vi "Init.vi"(0 "Experiment2D in":refnum<class "Experiment2D.lvclass">, 5 "Path":path=path "C:/Users/Sergei/Documents", 7 "Measurement2D.lvclass":refnum<class "Measurement2D.lvclass">, 9 "Data2D.lvclass":refnum<class "Data2D.lvclass">, 11 "error in (no error)":errorcluster) -> (4 "Experiment2D out":refnum<class "Experiment2D.lvclass">, 15 "error out":errorcluster)   [LabVIEW 2014, in "Experiment2D.lvclass"]
uses:
  Experiment2D.lvclass
  Measurement/Measurement2D/Measurement2D.lvclass
  Instrument/Instrument/Instrument.lvclass
  Data/Data2D/Data2D.lvclass
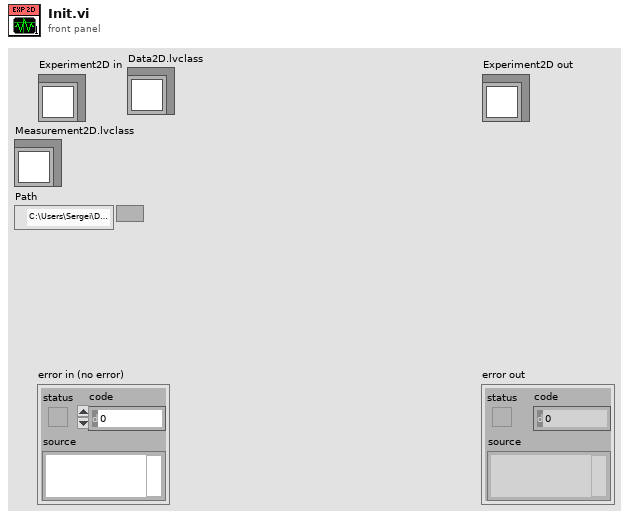
[diagram p1: front panel]
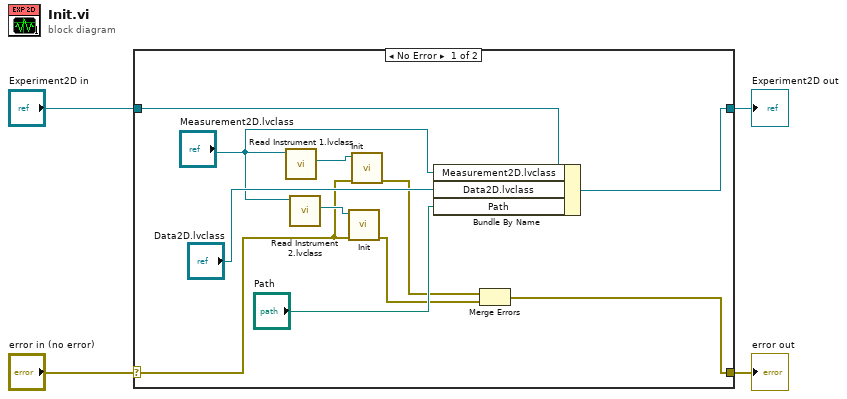
[diagram p0: block diagram]
diagram:
  n1 = case shown="No Error" "error in (no error)" {
    selector: "error in (no error)" -> [w8 w17]
    tunnel: [w5 w17] -> w3
    tunnel: [w14 w16] -> w1
    tunnel: "Experiment2D in" -> [w15 w16]
    frame No Error {
      n2 = call-dynamic "Read Instrument 1.lvclass.vi"("Measurement2D in"="Measurement2D.lvclass") -> ("Instrument.lvclass"=w12:refnum<class "Instrument.lvclass">)  [unwired: 8 in, 2 out]
      n3 = call-dynamic "Read Instrument 2.lvclass.vi"("Measurement2D in"="Measurement2D.lvclass") -> ("Instrument.lvclass"=w11:refnum<class "Instrument.lvclass">)  [unwired: 8 in, 2 out]
      n4 = call-dynamic "Init.vi"("error in (no error)"=w8, "Instrument in"=w11) -> ("error out"=w6:errorcluster)  [unwired: 8 in, 1 out]
      n5 = call-dynamic "Init.vi"("error in (no error)"=w8, "Instrument in"=w12) -> ("error out"=w7:errorcluster)  [unwired: 8 in, 1 out]
      n6 = Bundle By Name(cluster=w15, "Measurement2D.lvclass"="Measurement2D.lvclass", "Data2D.lvclass"="Data2D.lvclass", "Path"="Path") -> (w14:refnum<class "Experiment2D.lvclass">)
      n7 = Merge Errors(w7, w6) -> (w5:errorcluster)
    }
    frame Error {
    }
  }
  "error out" <- w3
  "Experiment2D out" <- w1
